vi "Tetris_DisplayLogicLoop.vi"   [LabVIEW 2018]
uses:
  <vilib>/Platform/TimedLoop/XDataNode/timing_clust.ctl
  <vilib>/Platform/TimedLoop/XDataNode/nitl_modes.ctl
  <vilib>/Platform/TimedLoop/XDataNode/wakeup.ctl
  <vilib>/rvi/Emulation/niFpgaSctlEmulationGetInTimedLoop.vi
  <vilib>/rvi/Emulation/niFpgaEmulationReportErrorSimple.vi
  <vilib>/rvi/Emulation/niFpgaGetClockAttributes.vi
  <vilib>/rvi/Emulation/niFpgaCriticalErrorInLSC.vi
  <vilib>/rvi/Emulation/niFpgaEmulationIsFPGAContextNoSignature.vi
  <vilib>/rvi/errors/niFpgaSetErrorForExecOnDevCompSimple.vi
  <vilib>/rvi/eio/common/nirviEmuReportErrorAndStop.vi
  <vilib>/rvi/DataTransferAndStorage/Container/Common/niFpgaContainerGetUniqueNameForEmu.vi
  <vilib>/rvi/FIFO/Fifo_Resource/nirvififoEmulationSetSize.vi
  <vilib>/rvi/FIFO/Fifo_Resource/nirviFifoEmulationQueueMgr.vi
  <instcachedir>/0/nirviFifoEmulationQueueMgr_E5CAEC123FF24DC58D834DCA3CDAA9B5.lvgen/nirviFifoEmulationQueueMgr_E5CAEC123FF24DC58D834DCA3CDAA9B5_002.vi
  <vilib>/rvi/FIFO/Fifo_Resource/nirvififoEmulationDetermineInputValidOut.vi
  <vilib>/rvi/FIFO/Fifo_Resource/nirvififoEmulationCreateLock.vi
  <vilib>/rvi/Emulation/niFpgaProcessEmulError.vi
  <vilib>/rvi/FIFO/Fifo_Resource/nirvififoEmulationObtainLock.vi
  <vilib>/rvi/FIFO/Fifo_Resource/nirvififoEmulationReleaseLock.vi
  <vilib>/rvi/occurrence/nirviWaitOnOccurrenceBase.vi
  <vilib>/rvi/errors/nirviReportUnexpectedCaseInternalError.vi
  <vilib>/rvi/errors/nirviReportUnexpectedCaseInternalError (U32).vi
  <vilib>/platform/TimedLoop/XDataNode/XDataNode.xnode
  <vilib>/rvi/DataTransferAndStorage/Container/XNode/niFpgaContainer.xnode
  <vilib>/rvi/FIFO/Fifo_Resource/nirvififoEmulationWrite.vi
  <vilib>/Platform/TimedLoop/XDataNode/XDNodeRunTimeDep.lvlib
types:
  T1 = typedef "XDNodeRunTimeDep.lvlib/timing_clust.ctl" = cluster{"Expected End [f-1]":u64, "Actual End [f-1]":u64, "Finished Late? [f-1]":bool, "Expected End [i-1]":u64, "Actual End [i-1]":u64, "Finished Late? [i-1]":bool, "Expected Start [i]":u64, "Actual Start [i]":u64, "Expected Start [f]":u64, "Actual Start [f]":u64, "Source Name":string, "Structure Name":string, "Period":i64, "Deadline":i64, "Offset":i64, "Start":i64, "Priority":i32, "Timeout":i32, "Mode":T2, "Wakeup Reason":T3, "Error":errorcluster, "Source Type":string, "Secondary Source Type":string, "Global End Time":u64, "Global Start Time":u64, "Frame Duration":u64, "Iteration Duration":u64, "Assigned CPU":i32, "I/O Scan Engine Mode":u32}
  T2 = typedef "XDNodeRunTimeDep.lvlib/nitl_modes.ctl" = enum32{"No Change", "Process missed periods, maintain original phase", "Discard missed periods, maintain original phase", "Process missed periods, ignore original phase", "Discard missed periods, ignore original phase"}
  T3 = typedef "XDNodeRunTimeDep.lvlib/wakeup.ctl" = enum32{"Normal", "Aborted", "Asynchronous wakeup", "Timing source error", "Timed loop error", "Timeout"}
  T4 = cluster{"left":i16, "top":i16, "right":i16, "bottom":i16}
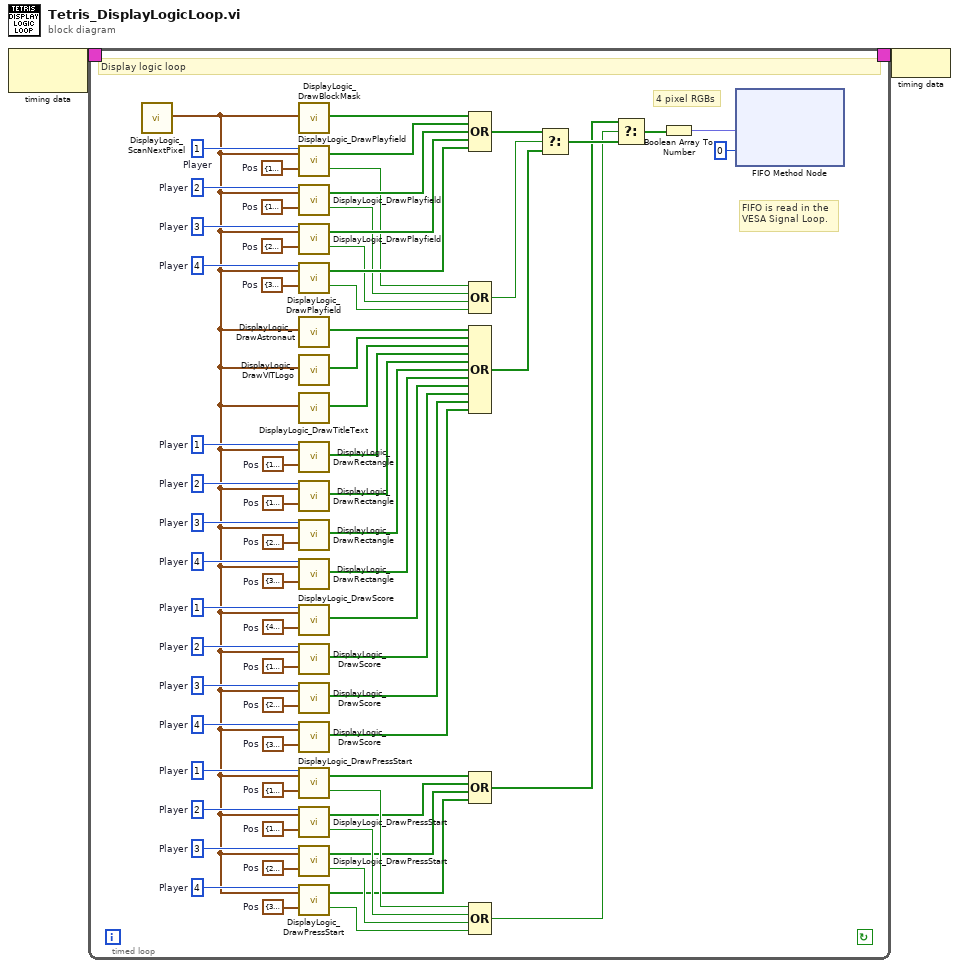
[diagram p0: block diagram]
diagram:
  n1 = node-c288() -> (w2:T1)  [unwired: 1 in]
  n2 = timed-loop {
    timing: w2 -> [_]
    timing-out: [_] -> w1
    stop <- _ continue-if-true
    w10 = T4 {"left"=333, "top"=1120, "right"=356, "bottom"=1151}  # Pos
    w11 = T4 {"left"=236, "top"=1120, "right"=259, "bottom"=1151}  # Pos
    w9 = T4 {"left"=140, "top"=1120, "right"=163, "bottom"=1151}  # Pos
    w8 = T4 {"left"=44, "top"=1120, "right"=67, "bottom"=1151}  # Pos
    w15 = u8 4  # Player
    w14 = u8 3  # Player
    w13 = u8 2  # Player
    w12 = u8 1  # Player
    w34 = T4 {"left"=304, "top"=556, "right"=384, "bottom"=617}  # Pos
    w35 = T4 {"left"=208, "top"=556, "right"=288, "bottom"=617}  # Pos
    w20 = T4 {"left"=112, "top"=556, "right"=192, "bottom"=617}  # Pos
    w33 = T4 {"left"=16, "top"=556, "right"=96, "bottom"=617}  # Pos
    w16 = u8 4  # Player
    w17 = u8 3  # Player
    w18 = u8 2  # Player
    w19 = u8 1  # Player
    w48 = T4 {"left"=304, "top"=1056, "right"=383, "bottom"=1088}  # Pos
    w47 = T4 {"left"=208, "top"=1056, "right"=287, "bottom"=1088}  # Pos
    w49 = T4 {"left"=112, "top"=1056, "right"=191, "bottom"=1088}  # Pos
    w50 = T4 {"left"=16, "top"=1056, "right"=95, "bottom"=1088}  # Pos
    w67 = T4 {"left"=304, "top"=384, "right"=383, "bottom"=1023}  # Pos
    w66 = T4 {"left"=208, "top"=384, "right"=287, "bottom"=1023}  # Pos
    w68 = T4 {"left"=112, "top"=384, "right"=191, "bottom"=1023}  # Pos
    w69 = T4 {"left"=16, "top"=384, "right"=95, "bottom"=1023}  # Pos
    w39 = u8 4  # Player
    w40 = u8 3  # Player
    w41 = u8 2  # Player
    w42 = u8 1  # Player
    w54 = u8 4  # Player
    w55 = u8 3  # Player
    w56 = u8 2  # Player
    w57 = u8 1  # Player
    # "4 pixel RGBs"
    # "FIFO is read in the\nVESA Signal Loop."
    # "Display logic loop"
    n3 = call "DisplayLogic_ScanNextPixel.vi"() -> ("ActivePixel"=w7:cluster{"h_pixel":i16, "v_pixel":i16})  [unwired: 19 in]
    n4 = call "DisplayLogic_DrawBlockMask.vi"("ActivePixel"=w7) -> ("PixelData"=w37:bool[])  [unwired: 18 in]
    n5 = call "DisplayLogic_DrawPlayfield.vi"("Player"=w57, "ActivePixel"=w7, "PlayfieldPosition"=w69) -> ("PixelData"=w65:bool[], "Draw"=w61:bool)  [unwired: 15 in]
    n6 = call "DisplayLogic_DrawPlayfield.vi"("Player"=w56, "ActivePixel"=w7, "PlayfieldPosition"=w68) -> ("PixelData"=w64:bool[], "Draw"=w60:bool)  [unwired: 15 in]
    n7 = call "DisplayLogic_DrawPlayfield.vi"("Player"=w55, "ActivePixel"=w7, "PlayfieldPosition"=w66) -> ("PixelData"=w63:bool[], "Draw"=w59:bool)  [unwired: 15 in]
    n8 = call "DisplayLogic_DrawPlayfield.vi"("Player"=w54, "ActivePixel"=w7, "PlayfieldPosition"=w67) -> ("PixelData"=w62:bool[], "Draw"=w58:bool)  [unwired: 15 in]
    n9 = call "DisplayLogic_DrawAstronaut.vi"("ActivePixel"=w7) -> ("PixelData"=w51:bool[])  [unwired: 18 in]
    n10 = call "DisplayLogic_DrawVITLogo.vi"("ActivePixel"=w7) -> ("PixelData"=w53:bool[])  [unwired: 18 in]
    n11 = call "DisplayLogic_DrawTitleText.vi"("ActivePixel"=w7) -> ("PixelData"=w52:bool[])  [unwired: 18 in]
    n12 = call "DisplayLogic_DrawRectangle.vi"("Player"=w42, "ActivePixel"=w7, "RectanglePosition"=w50) -> ("PixelData"=w43:bool[])  [unwired: 16 in]
    n13 = call "DisplayLogic_DrawRectangle.vi"("Player"=w41, "ActivePixel"=w7, "RectanglePosition"=w49) -> ("PixelData"=w44:bool[])  [unwired: 16 in]
    n14 = call "DisplayLogic_DrawRectangle.vi"("Player"=w40, "ActivePixel"=w7, "RectanglePosition"=w47) -> ("PixelData"=w45:bool[])  [unwired: 16 in]
    n15 = call "DisplayLogic_DrawRectangle.vi"("Player"=w39, "ActivePixel"=w7, "RectanglePosition"=w48) -> ("PixelData"=w46:bool[])  [unwired: 16 in]
    n16 = call "DisplayLogic_DrawScore.vi"("Player"=w12, "ActivePixel"=w7, "ScorePosition"=w8) -> ("PixelData"=w6:bool[])  [unwired: 16 in]
    n17 = call "DisplayLogic_DrawScore.vi"("Player"=w13, "ActivePixel"=w7, "ScorePosition"=w9) -> ("PixelData"=w5:bool[])  [unwired: 16 in]
    n18 = call "DisplayLogic_DrawScore.vi"("Player"=w14, "ActivePixel"=w7, "ScorePosition"=w11) -> ("PixelData"=w4:bool[])  [unwired: 16 in]
    n19 = call "DisplayLogic_DrawScore.vi"("Player"=w15, "ActivePixel"=w7, "ScorePosition"=w10) -> ("PixelData"=w3:bool[])  [unwired: 16 in]
    n20 = call "DisplayLogic_DrawPressStart.vi"("Player"=w19, "ActivePixel"=w7, "PressStartPos"=w33) -> ("PixelData"=w25:bool[], "Draw"=w30:bool)  [unwired: 15 in]
    n21 = call "DisplayLogic_DrawPressStart.vi"("Player"=w18, "ActivePixel"=w7, "PressStartPos"=w20) -> ("PixelData"=w24:bool[], "Draw"=w29:bool)  [unwired: 15 in]
    n22 = call "DisplayLogic_DrawPressStart.vi"("Player"=w17, "ActivePixel"=w7, "PressStartPos"=w35) -> ("PixelData"=w23:bool[], "Draw"=w28:bool)  [unwired: 15 in]
    n23 = call "DisplayLogic_DrawPressStart.vi"("Player"=w16, "ActivePixel"=w7, "PressStartPos"=w34) -> ("PixelData"=w22:bool[], "Draw"=w27:bool)  [unwired: 15 in]
    n24 = Compound Arithmetic op=OR ("OR")(w37, w65, w64, w63, w62) -> (w36:bool[])
    n25 = Compound Arithmetic op=OR ("OR")(w61, w60, w59, w58) -> (w38:bool)
    n26 = Compound Arithmetic op=OR ("OR")(w51, w53, w52, w43, w44, w45, w46, w6, w5, w4, w3) -> (w70:bool[])
    n27 = Compound Arithmetic op=OR ("OR")(w25, w24, w23, w22) -> (w21:bool[])
    n28 = Compound Arithmetic op=OR ("OR")(w30, w29, w28, w27) -> (w26:bool)
    n29 = Select(t=w36, s=w38, f=w70) -> (s? t:f=w32:bool[])
    n30 = Select(t=w21, s=w26, f=w32) -> (s? t:f=w31:bool[])
    n31 = Boolean Array To Number(Boolean array=w31) -> (number=w71:fxp<+,12,12>)
    n32 = xnode ("FIFO Method Node")("Element"=w71, "Timeout"=0) -> ()  [unwired: 1 in, 2 out]
  }
  n33 = node-c288(w1) -> ()
